vi "CAN Reset.vi"(8 "错误输入（无错误）":errorcluster, 11 "Channel in":u16) -> (0 "错误输出":errorcluster, 2 "Channel out":u16, 3 "TCANStatus":T1 items=["PCAN_ERROR_OK"=0, "PCAN_ERROR_XMTFULL"=1, "PCAN_ERROR_OVERRUN"=2, "PCAN_ERROR_BUSLIGHT"=4, "PCAN_ERROR_BUSHEAVY"=8, "PCAN_ERROR_BUSPASSIVE"=262144, "PCAN_ERROR_BUSOFF"=16, "PCAN_ERROR_QRCVEMPTY"=32, "PCAN_ERROR_QOVERRUN"=64, "PCAN_ERROR_QXMTFULL"=128, "PCAN_ERROR_REGTEST"=256, "PCAN_ERROR_NODRIVER"=512, "PCAN_ERROR_HWINUSE"=1024, "PCAN_ERROR_NETINUSE"=2048, "PCAN_ERROR_ILLHW"=5120, "PCAN_ERROR_ILLNET"=6144, "PCAN_ERROR_ILLCLIENT"=7168, "PCAN_ERROR_RESOURCE"=8192, "PCAN_ERROR_ILLPARAMTYPE"=16384, "PCAN_ERROR_ILLPARAMVAL"=32768, "PCAN_ERROR_UNKNOWN"=65536, "PCAN_ERROR_ILLDATA"=131072, "PCAN_ERROR_CAUTION"=33554432, "PCAN_ERROR_INITIALIZE"=67108864, "PCAN_ERROR_ILLOPERATION"=134217728])   [LabVIEW 2020, in "PCANBasic.lvlib"]
doc: "TPCANStatus __stdcall CAN_Reset(\n TPCANHandle Channel);"
uses:
  <userlib>/PCANBasic/PCANBasic.lvlib
  <userlib>/PCANBasic/ctl/TPCANStatus.ctl
  <userlib>/PCANBasic/PCANBasic.dll
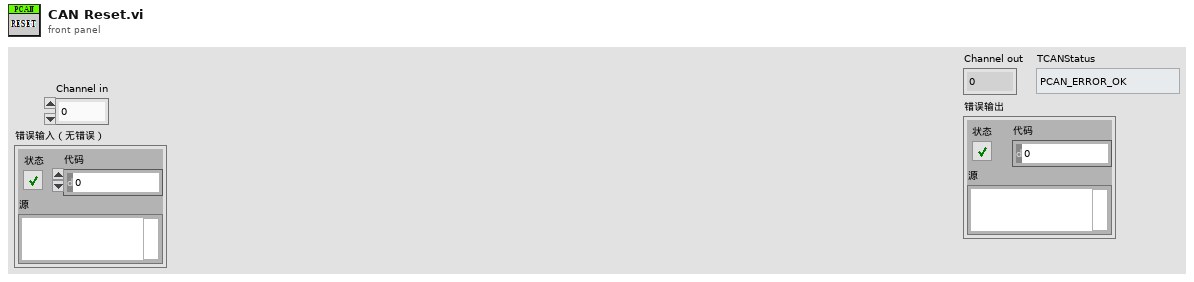
[diagram p1: front panel]
types:
  T1 = typedef "PCANBasic.lvlib/TPCANStatus.ctl" = u32
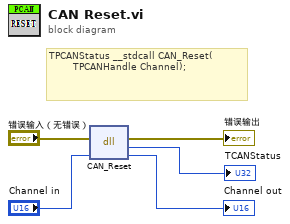
[diagram p0: block diagram]
diagram:
  # "TPCANStatus __stdcall CAN_Reset(\n        TPCANHandle Channel);"
  n1 = dll-call lib="D:/Program Files (x86)/National Instruments/LabVIEW 2020/user.lib/PCANBasic/PCANBasic.dll" fn="CAN_Reset"(error in="错误输入（无错误）", "Channel"="Channel in") -> (error out=→"错误输出":errorcluster, "返回类型"=→"TCANStatus":u32, "Channel"=→"Channel out":u16)  [unwired: 2 in, 1 out]
